vi "模块配置写入.vi"(8 "error in (no error)":errorcluster caption="错误输入（无错误）") -> (0 "错误输出":errorcluster)   [LabVIEW 2016, in "斯坦道通用流路CODmn.lvlib"]
uses:
  <vilib>/Utility/config.llb/NI_LVConfig.lvlib
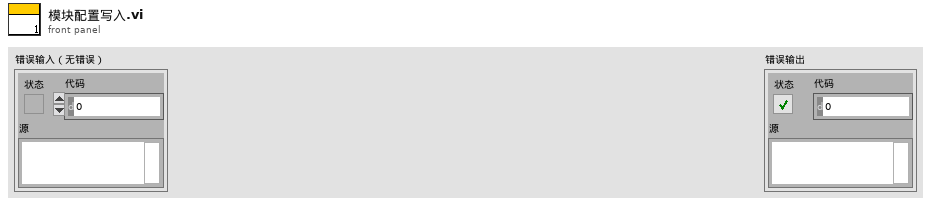
[diagram p1: front panel]
types:
  T1 = typedef "NI_LVConfig.lvlib/Config Data RefNum.ctl" = refnum<k1>
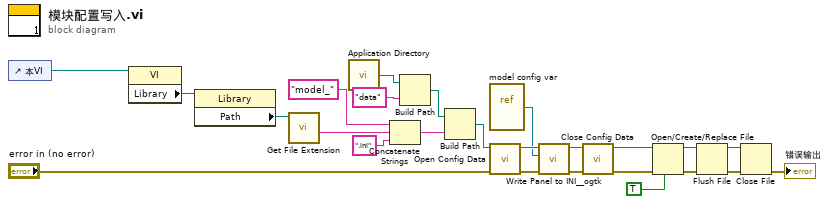
[diagram p0: block diagram]
diagram:
  n1 = control-ref of="本VI"() -> (w7:refnum<vi>)
  n2 = property class="VI"(reference=w7) -> ("Library"=w8:refnum<vi>)  [unwired: 1 in, 2 out]
  n3 = property class="Library"(reference=w8) -> ("Path"=w2:path)  [unwired: 1 in, 2 out]
  n4 = call <vilib>:"Get File Extension.vi"("file"=w2) -> ("filename without extension"=w1:string)  [unwired: 6 in, 4 out]
  n5 = call <vilib>:"Application Directory.vi"() -> ("Application Directory"=w10:path)
  n6 = Concatenate Strings("model_" ("字符串"), w1, ".ini" ("字符串")) -> (w6:string)
  n7 = Build Path(base path=w10, name or relative path="data" ("名称或相对路径")) -> (appended path=w9:path)
  n8 = Build Path(base path=w9, name or relative path=w6) -> (appended path=w3:path)
  n9 = vi-ref "model config var.vi"() -> (w24:refnum<vi>)
  n10 = call <vilib>:"Open Config Data.vi"("error in (no error)"="error in (no error)", "configuration file path"=w3) -> ("error out"=w22:errorcluster, "refnum"=w25:T1)  [unwired: 7 in, 1 out]
  n11 = call <userlib>:"Write Panel to INI__ogtk.vi"("error in (no error)"=w22, "VI ref"=w24, "refnum"=w25) -> ("error out"=w21:errorcluster, "refnum out"=w23:T1)  [unwired: 7 in]
  n12 = call <vilib>:"Close Config Data.vi"("error in (no error)"=w21, "refnum"=w23) -> ("error out"=w16:errorcluster, "file path"=w15:path)  [unwired: 8 in]
  n13 = Open/Create/Replace File(file path (use dialog)=w15, error in=w16, disable buffering (F)=TRUE ("禁用缓存(F)")) -> (refnum out=w19:refnum<file>, error out=w20:errorcluster)  [unwired: 3 in, 1 out]
  n14 = Flush File(refnum=w19, error in=w20) -> (refnum out=w18:refnum<file>, error out=w17:errorcluster)
  n15 = Close File(refnum=w18, error in=w17) -> (error out=→"错误输出":errorcluster)  [unwired: 1 out]
